vi "Set Out_Data.vi"(8 "error in (no error)":errorcluster caption="entrée d'erreur (pas d'erreur)", 10 "Out_Data":T1, 11 "Firebase Packaging en entrée":refnum<class "Firebase Packaging.lvclass">) -> (0 "error out":errorcluster caption="sortie d'erreur", 3 "Firebase Packaging en sortie":refnum<class "Firebase Packaging.lvclass">)   [LabVIEW 2020, in "Library Instrument & Equipement.lvlib" / "Library FireBase.lvlib" / "Firebase Packaging.lvclass"]
uses:
  Firebase Packaging.lvclass
  Firebase Packaging.lvclass/Firebase Packaging.ctl
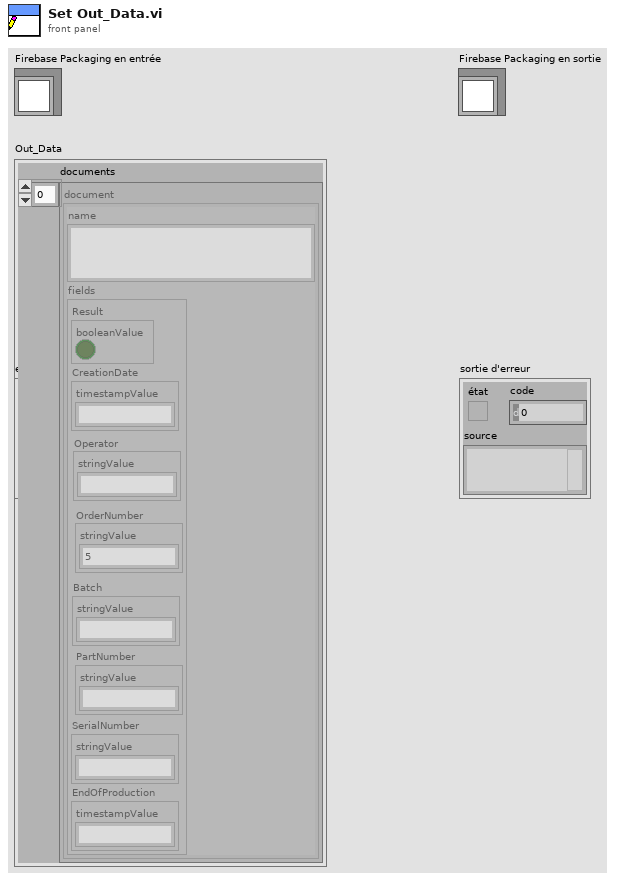
[diagram p1: front panel]
types:
  T1 = cluster{"documents":cluster{"name":string, "fields":cluster{"Result":cluster{"booleanValue":bool}, "CreationDate":cluster{"timestampValue":string}, "Batch":cluster{"stringValue":string}, "SerialNumber":cluster{"stringValue":string}, "EndOfProduction":cluster{"timestampValue":string}, "PartNumber":cluster{"stringValue":string}, "OrderNumber":cluster{"stringValue":string}, "Operator":cluster{"stringValue":string}}}[]}
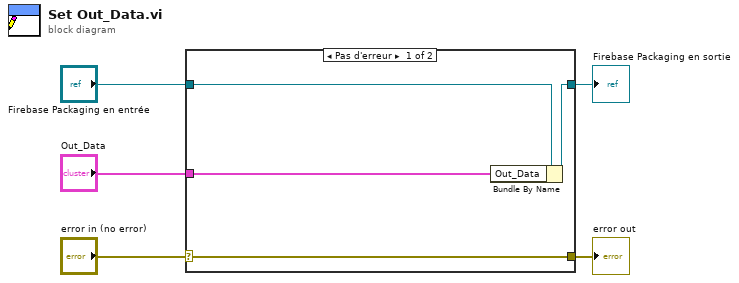
[diagram p0: block diagram]
diagram:
  n1 = case shown="Pas d'erreur" "error in (no error)" {
    selector: "error in (no error)" -> [w9 w10]
    tunnel: [w9 w10] -> w4
    tunnel: [w7 w11] -> w2
    tunnel: "Firebase Packaging en entrée" -> [w8 w11]
    tunnel: "Out_Data" -> [w6 _]
    frame No Error {
      n2 = Bundle By Name(cluster=w8, "Out_Data"=w6) -> (w7:refnum<class "Firebase Packaging.lvclass">)
    }
    frame Error {
    }
  }
  "error out" <- w4
  "Firebase Packaging en sortie" <- w2
